vi "KDH_EX3Task3_1-19-17.vi"() -> ()   [LabVIEW 2014, in "Harris_MacMaster_4th_LEGORobotics_11-29-16.lvrbt"]
uses:
  Harris_MacMaster_4th_LEGORobotics_11-29-16.lvrbt
panel:
  out "Moving Average":dbl
  in  "stop":bool
  out "Random Number":dbl
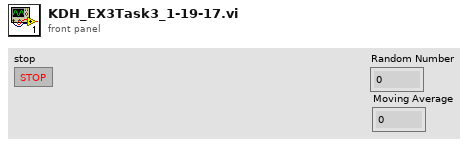
[diagram p1: front panel]
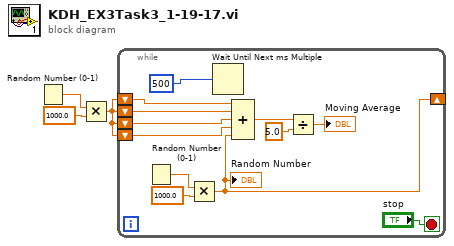
[diagram p0: block diagram]
diagram:
  n1 = Random Number (0-1)() -> (number: 0 to 1=w2:dbl)
  n2 = Multiply(x=w2, y=1000.0) -> (x*y=w1:dbl)
  n3 = while {
    shift-right: [w5] -> _
    shift-left: w1 -> [w12]
    shift-left: w1 -> [w11]
    shift-left: w1 -> [w10]
    shift-left: w1 -> [w9]
    stop <- "stop" stop-if-true
    n4 = Random Number (0-1)() -> (number: 0 to 1=w14:dbl)
    n5 = Multiply(x=w14, y=1000.0) -> (x*y=w5:dbl)
    "Random Number" <- w5
    n6 = Wait Until Next ms Multiple(millisecond multiple=u32 500) -> ()  [unwired: 1 out]
    n7 = Compound Arithmetic op=ADD(w12, w11, w10, w9, w5) -> (w7:dbl)
    n8 = Divide(x=w7, y=5.0) -> (x/y=→"Moving Average":dbl)
  }
